vi "Destroy OOB Communications.vi"(8 "error in (no error)":errorcluster, 11 "CIFTemplatePlugin in":refnum<class "TemplatePlugin.lvclass">) -> (0 "error out":errorcluster, 3 "CIFTemplatePlugin out":refnum<class "TemplatePlugin.lvclass">)   [LabVIEW 2021, in "TemplatePlugin.lvclass"]
uses:
  TemplatePlugin.lvclass
  TemplatePlugin.lvclass/TemplatePlugin.ctl
  OOB/OOB_Rx/TemplateOOB_Rx.lvclass
  OOB/OOB_Tx/TemplateOOB_Tx.lvclass
  CIF-LVCore/src/CIFUtilities/CIFOutOfBand/CIFOutOfBand.lvclass
  D:/dev/CIF-LVCore/src/CIFUtilities/CIFOutOfBand/CIFOutOfBand.lvclass
  D:/dev/Plugins/Template/OOB/OOB_Rx/TemplateOOB_Rx.lvclass
  D:/dev/Plugins/Template/OOB/OOB_Tx/TemplateOOB_Tx.lvclass
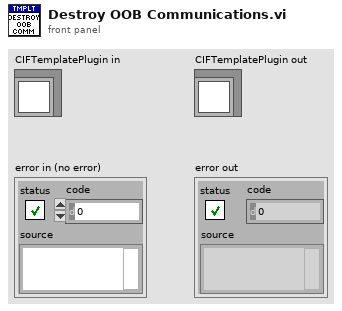
[diagram p1: front panel]
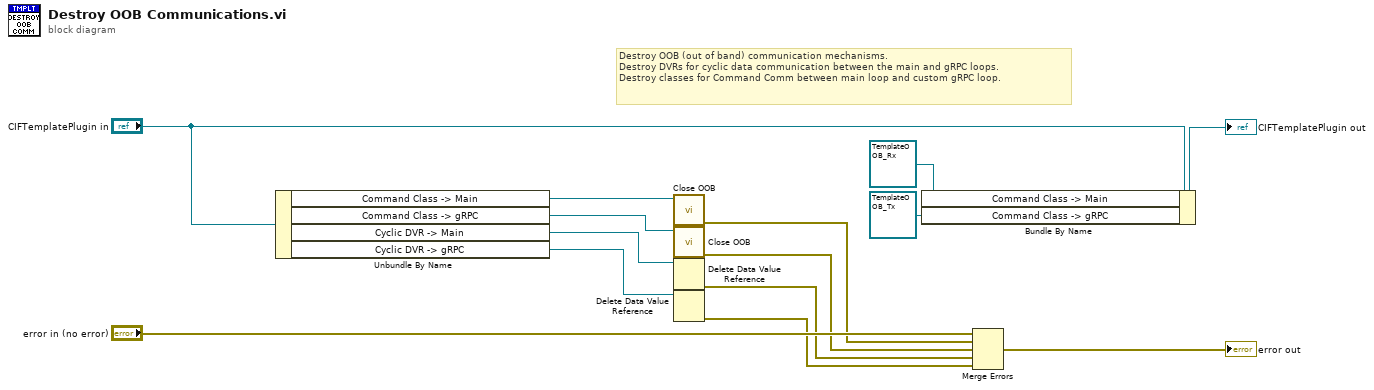
[diagram p0: block diagram]
diagram:
  # "Destroy OOB (out of band) communication mechanisms.\nDestroy DVRs for cyclic data communication between the main and gRPC loops. \nDestroy classes for Command Comm between main loop and custom gRPC loop."
  n1 = Unbundle By Name("CIFTemplatePlugin in") -> ("Command Class -> Main"=w11:refnum<class "TemplateOOB_Rx.lvclass">, "Command Class -> gRPC"=w7:refnum<class "TemplateOOB_Tx.lvclass">, "Cyclic DVR -> Main"=w6:refnum<data-value>, "Cyclic DVR -> gRPC"=w8:refnum<data-value>)
  n2 = call "Close OOB.vi"("OOB in"=w11) -> ("error out"=w2:errorcluster)  [unwired: 10 in]
  n3 = call "Close OOB.vi"("OOB in"=w7) -> ("error out"=w3:errorcluster)  [unwired: 10 in]
  n4 = Delete Data Value Reference(data value reference=w6) -> (error out=w4:errorcluster)  [unwired: 1 in, 1 out]
  n5 = Delete Data Value Reference(data value reference=w8) -> (error out=w5:errorcluster)  [unwired: 1 in, 1 out]
  n6 = Bundle By Name(cluster="CIFTemplatePlugin in", "Command Class -> Main"=refnum<class "TemplateOOB_Rx.lvclass"> refnum ("CutomOOB_Rx out"), "Command Class -> gRPC"=refnum<class "TemplateOOB_Tx.lvclass"> refnum ("CutomOOB_Tx out")) -> (→"CIFTemplatePlugin out":refnum<class "TemplatePlugin.lvclass">)
  n7 = Merge Errors("error in (no error)", w2, w3, w4, w5) -> (→"error out":errorcluster)
